vi "subpull5.vi"() -> ()   [LabVIEW 2011]
panel:
  out "Output Baseband IQ":cdb[](array[numeric])
  in  "Input Baseband IQ":cdb[](array[numeric])
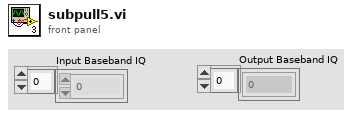
[diagram p1: front panel]
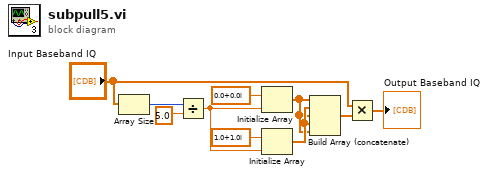
[diagram p0: block diagram]
diagram:
  n1 = Array Size(array="Input Baseband IQ") -> (size(s)=w10:i32)
  n2 = Divide(x=w10, y=5.0) -> (x/y=w7:dbl)
  n3 = Initialize Array(cdb 0.0+0.0i ("element"), w7) -> (w4:cdb[])
  n4 = Initialize Array(cdb 1.0+1.0i ("element"), w7) -> (w5:cdb[])
  n5 = Build Array (concatenate)(w4, w5, w4, w5, w4) -> (w3:cdb[])
  n6 = Multiply(x="Input Baseband IQ", y=w3) -> (x*y=→"Output Baseband IQ":cdb[])
